vi "ScanDone.vi"(8 "error in (no error)":errorcluster, 11 "Camera_Controller in":refnum<class "Camera_Controller.lvclass">) -> (0 "error out":errorcluster, 3 "Camera_Controller out":refnum<class "Camera_Controller.lvclass">)   [LabVIEW 2023, in "Camera_Controller.lvlib" / "Camera_Controller.lvclass"]
uses:
  Camera_Controller.lvclass
  Camera_Controller.lvclass/Camera_Controller.ctl
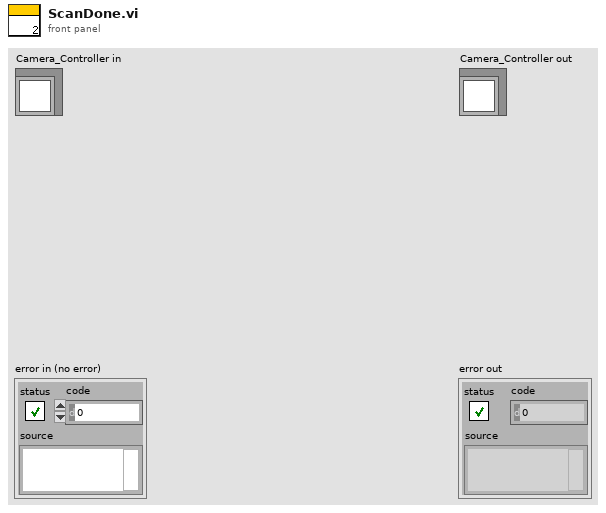
[diagram p1: front panel]
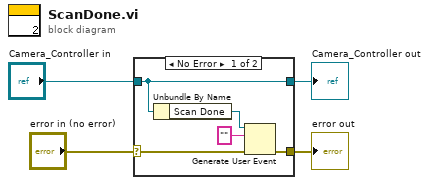
[diagram p0: block diagram]
diagram:
  n1 = case shown="No Error" "error in (no error)" {
    selector: "error in (no error)" -> [w5 w11]
    tunnel: [w6 w11] -> w2
    tunnel: [w9 w10] -> w1
    tunnel: "Camera_Controller in" -> [w9 w10]
    frame No Error {
      n2 = Unbundle By Name(w9) -> ("Scan Done"=w8:refnum<user-event>)
      n3 = Generate User Event(user event=w8, event data cluster="" ("event data"), error in=w5) -> (error out=w6:errorcluster)  [unwired: 1 in, 1 out]
    }
    frame Error {
    }
  }
  "error out" <- w2
  "Camera_Controller out" <- w1
